vi "WriteVariableI32.vi"(6 "ns":i32=2, 8 "error in (no error)":errorcluster, 9 "value":i32, 10 "variable_node":string, 11 "Server in":refnum<class "Server.lvclass">) -> (0 "error out":errorcluster, 3 "Server out":refnum<class "Server.lvclass">)   [LabVIEW 2017, in "opcua.lvlib" / "Server.lvclass"]
uses:
  Server.lvclass
  Server.lvclass/Server.ctl
  opcua32.dll
  opcua.lvlib
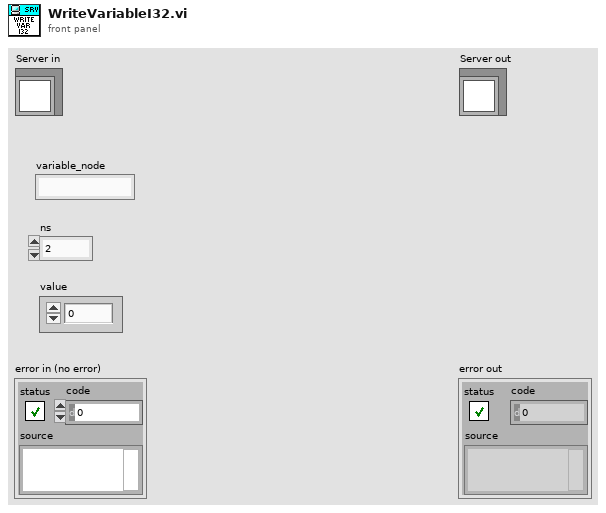
[diagram p1: front panel]
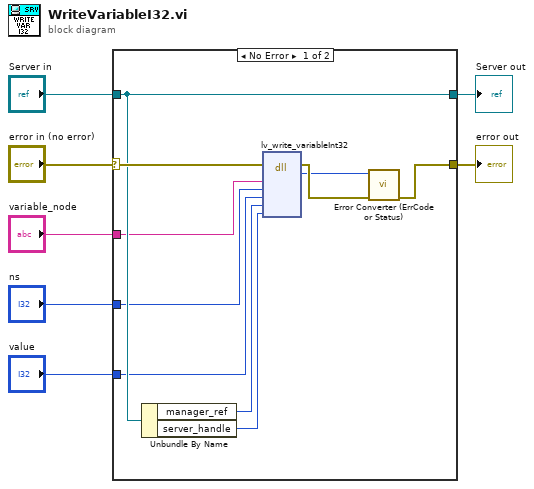
[diagram p0: block diagram]
diagram:
  n1 = case shown="No Error" "error in (no error)" {
    selector: "error in (no error)" -> [w16 w18]
    tunnel: [w9 w18] -> w6
    tunnel: [w14 w19] -> w4
    tunnel: "Server in" -> [w14 w19]
    tunnel: "value" -> [w13 _]
    tunnel: "variable_node" -> [w12 _]
    tunnel: "ns" -> [w11 _]
    frame No Error {
      n2 = Unbundle By Name(w14) -> ("manager_ref"=w17:u64, "server_handle"=w15:u64)
      n3 = dll-call lib="C:/Users/Andrey/Desktop/opcua-labview/opcua-lvlib/opcua*.dll" fn="lv_write_variableInt32"(error in=w16, "variable_node"=w12, "ns"=w11, "value"=w13, "manager"=w17, "handle"=w15) -> (error out=w10:errorcluster, "return type"=w8:i32)  [unwired: 7 in, 1 out]
      n4 = call "Error Converter (ErrCode or Status).vi"("error in (no error)"=w10, "error code"=w8) -> ("error out"=w9:errorcluster)  [unwired: 9 in]
    }
    frame Error {
    }
  }
  "error out" <- w6
  "Server out" <- w4
